vi "lsignKey.vi"(0 "HGF_GPG":refnum<class "HGF_GPG.lvclass">, 1 "options file":path, 2 "keyringfile":path, 3 "Sec keyringfile":path, 4 "id2sign":string, 5 "error in (no error)":errorcluster, 6 "key-id":string, 7 "password":string, 8 "Trust DB":path) -> (10 "dup Trust DB":path, 11 "standard output":string, 13 "data error?":bool, 14 "dup HGF_GPG":refnum<class "HGF_GPG.lvclass">, 15 "dup options file":path, 16 "dup keyringfile":path, 17 "dup Sec keyringfile":path, 18 "standard error":string, 19 "error out":errorcluster)   [LabVIEW 2012, in "HGF_GPG.lvlib" / "HGF_GPG.lvclass"]
doc: "Sign a GPG-Key for local use. This signature will not be exported with the key, or updated to a server."
uses:
  HGF_GPG.lvclass
  HGF_GPG.lvclass/HGF_GPG.ctl
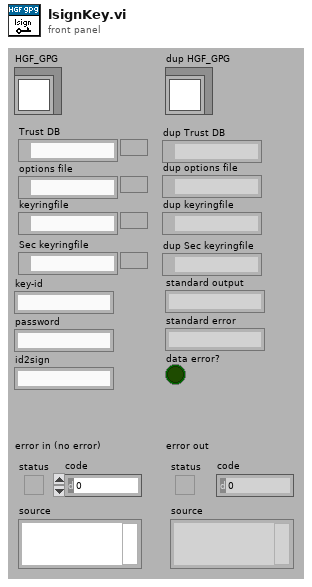
[diagram p1: front panel]
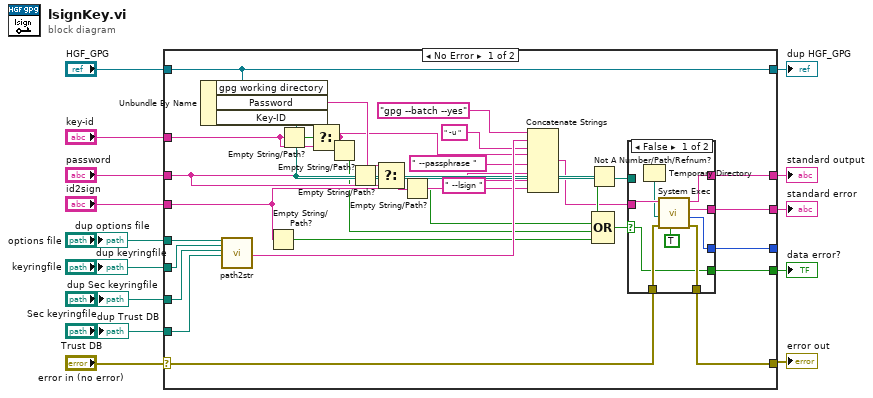
[diagram p0: block diagram]
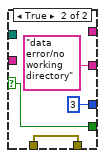
[diagram p2: hidden frame]
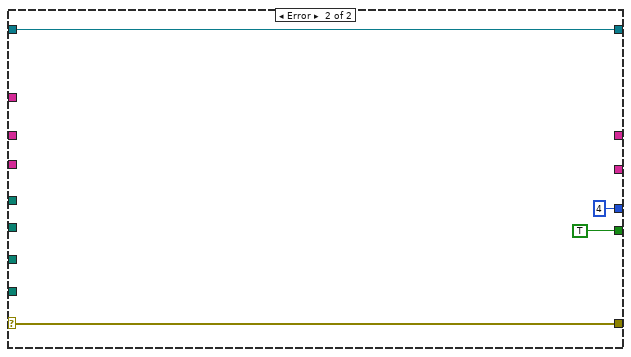
[diagram p3: hidden frame]
diagram:
  n1 = case shown="No Error" "error in (no error)" {
    selector: "error in (no error)" -> [w40 w63]
    tunnel: [w39 w63] -> w8
    tunnel: [w45 w62] -> w13
    tunnel: "HGF_GPG" -> [w45 w62]
    tunnel: [w38 4 ("return code")] -> _
    tunnel: [w37 _] -> w6
    tunnel: [w36 _] -> w7
    tunnel: "key-id" -> [w20 _]
    tunnel: "password" -> [w33 _]
    tunnel: "id2sign" -> [w26 _]
    tunnel: [w19 TRUE] -> w9
    tunnel: "keyringfile" -> [w18 _]
    tunnel: "options file" -> [w17 _]
    tunnel: "Sec keyringfile" -> [w16 _]
    tunnel: "Trust DB" -> [w15 _]
    frame No Error {
      n2 = Unbundle By Name(w45) -> ("gpg working directory"=w41:path, "Password"=w34:string, "Key-ID"=w21:string)
      n3 = call "path2str.vi"("options file"=w17, "keyringfile"=w18, "Sec keyringfile"=w16, "Trust DB"=w15) -> ("opt/keyr/seckeyr/trusdb"=w46:string)  [unwired: 2 in, 13 out]
      n4 = Empty String/Path?(string/path=w26) -> (empty?=w23:bool)
      n5 = Empty String/Path?(string/path=w20) -> (empty?=w44:bool)
      n6 = Select(t=w21, s=w44, f=w20) -> (s? t:f=w30:string)
      n7 = Empty String/Path?(string/path=w30) -> (empty?=w24:bool)
      n8 = Empty String/Path?(string/path=w33) -> (empty?=w35:bool)
      n9 = Select(t=w34, s=w35, f=w33) -> (s? t:f=w28:string)
      n10 = Empty String/Path?(string/path=w28) -> (empty?=w25:bool)
      n11 = Concatenate Strings("gpg --batch --yes", w46, " -u " ("string"), w30, " --passphrase " ("string"), w28, " --lsign " ("string"), w26) -> (w22:string)
      n12 = Not A Number/Path/Refnum?(number/path/refnum=w41) -> (NaN/Path/Refnum?=w43:bool)
      n13 = Compound Arithmetic op=OR(w43, w25, w24, w23) -> (w42:bool)
      n14 = case shown="False" w42 {
        selector: w42 -> [w48 w56]
        tunnel: w40 -> [w54 w59]
        tunnel: [w53 w59] -> w39
        tunnel: w41 -> [_ _]
        tunnel: [w52 _] -> w36
        tunnel: [w51 "data error/no working directory" ("standard error")] -> w37
        tunnel: [w50 3 ("return code")] -> w38
        tunnel: w22 -> [w49 _]
        tunnel: [w48 w56] -> w19
        frame False {
          n15 = Temporary Directory() -> (w47:path)
          n16 = call <vilib>:"System Exec.vi"("run minimized? (F)"=TRUE, "error in (no error)"=w54, "working directory"=w47, "command line"=w49) -> ("error out"=w53:errorcluster, "return code"=w50:i32, "standard error"=w51:string, "standard output"=w52:string)  [unwired: 2 in, 2 out]
        }
        frame True {
        }
      }
    }
    frame Error {
    }
  }
  "error out" <- w8
  "dup HGF_GPG" <- w13
  "data error?" <- w9
  "standard output" <- w7
  "standard error" <- w6
  "dup options file" <- "options file"
  "dup keyringfile" <- "keyringfile"
  "dup Sec keyringfile" <- "Sec keyringfile"
  "dup Trust DB" <- "Trust DB"
